vi "SimpleDownsample5.vi"(7 "reset":bool, 10 "Data in 1":fxp<+/-,16,14>, 11 "Data in 0":fxp<+/-,16,14>) -> (0 "data valid":bool, 3 "Data out":fxp<+/-,16,14>)   [LabVIEW 2013]
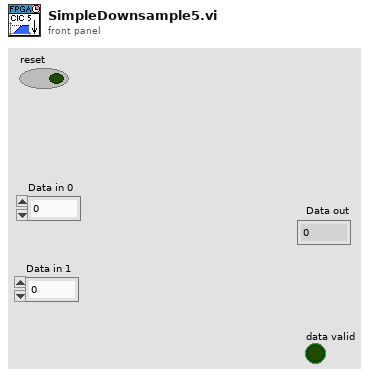
[diagram p1: front panel]
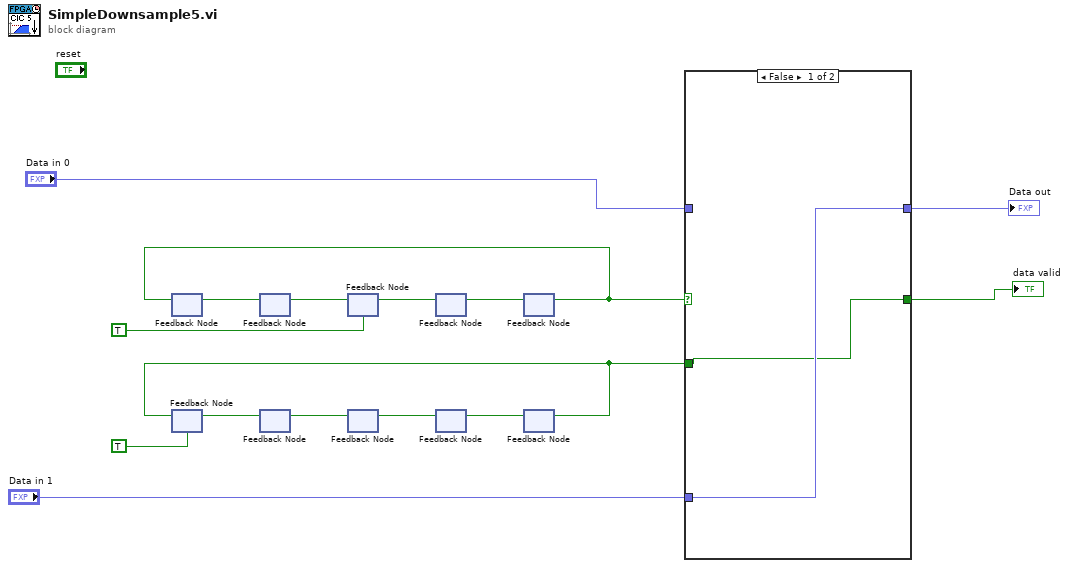
[diagram p0: block diagram]
diagram:
  n1 = feedback #1() -> (w16:bool)  [unwired: 1 in]
  n2 = feedback #2(TRUE) -> (w9:bool)
  n3 = feedback #3() -> (w15:bool)  [unwired: 1 in]
  n4 = feedback-in #3(w16) -> ()
  n5 = feedback #4() -> (w10:bool)  [unwired: 1 in]
  n6 = feedback-in #4(w9) -> ()
  n7 = feedback #5(TRUE) -> (w14:bool)
  n8 = feedback-in #5(w15) -> ()
  n9 = feedback #6() -> (w11:bool)  [unwired: 1 in]
  n10 = feedback-in #6(w10) -> ()
  n11 = feedback #7() -> (w13:bool)  [unwired: 1 in]
  n12 = feedback-in #7(w14) -> ()
  n13 = feedback #8() -> (w12:bool)  [unwired: 1 in]
  n14 = feedback-in #8(w11) -> ()
  n15 = feedback #9() -> (w6:bool)  [unwired: 1 in]
  n16 = feedback-in #1(w6) -> ()
  n17 = feedback-in #9(w13) -> ()
  n18 = feedback #10() -> (w2:bool)  [unwired: 1 in]
  n19 = feedback-in #2(w2) -> ()
  n20 = feedback-in #10(w12) -> ()
  n21 = case shown="False" w6 {
    selector: w6 -> [_ w19]
    tunnel: "Data in 0" -> [_ w20]
    tunnel: [w18 w20] -> w4
    tunnel: [w17 w19] -> w3
    tunnel: w2 -> [w17 _]
    tunnel: "Data in 1" -> [w18 _]
    frame False {
    }
    frame True {
    }
  }
  "Data out" <- w4
  "data valid" <- w3
